vi "WFS Get Spot Dia Statistics.vi"(8 "error in (no error)":errorcluster {"code" format="%.0x"}, 11 "instrument handle":refnum<visa-resource-name>) -> (0 "error out":errorcluster {"code" format="%.0x"}, 1 "Max":dbl, 2 "Min":dbl, 3 "instrument handle out":refnum<visa-resource-name>, 4 "Mean":dbl)   [LabVIEW 2020]
doc: "This VI calculates statistic parameters of the wavefront calculated in WFS Calc Wavefront.vi.\n\nNote: WFS Calc Wavefront.vi is required to run prior to this VI.\nThis VI is not available in Highspeed Mode!"
uses:
  WFS_32.dll
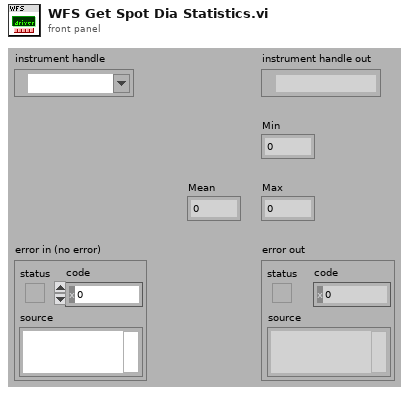
[diagram p1: front panel]
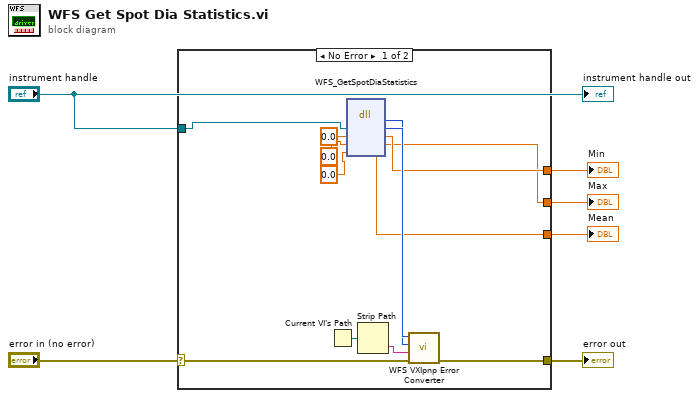
[diagram p0: block diagram]
diagram:
  n1 = case shown="No Error" "error in (no error)" {
    selector: "error in (no error)" -> [w14 w20]
    tunnel: [w13 w20] -> w6
    tunnel: "instrument handle" -> [w18 _]
    tunnel: [w11 _] -> w3
    tunnel: [w9 _] -> w2
    tunnel: [w7 _] -> w1
    frame No Error {
      n2 = Current VI's Path() -> (path=w19:path)
      n3 = dll-call lib="WFS_*.*" fn="WFS_GetSpotDiaStatistics"("Instrument Handle"=w18, "Min"=0.0, "Max"=0.0, "Mean"=0.0) -> (w16:i32, "Instrument Handle"=w17:u32, "Min"=w11:dbl, "Max"=w9:dbl, "Mean"=w7:dbl)  [unwired: 3 in, 2 out]
      n4 = Strip Path(path=w19) -> (name=w15:string)  [unwired: 1 out]
      n5 = call "WFS VXIpnp Error Converter.vi"("error in (no error)"=w14, "Name Of VI (\"\")"=w15, "CVI Error Code (0)"=w16, "instrument handle"=w17) -> ("error out"=w13:errorcluster)  [unwired: 6 in, 1 out]
    }
    frame Error {
    }
  }
  "error out" <- w6
  "Min" <- w3
  "Max" <- w2
  "Mean" <- w1
  "instrument handle out" <- "instrument handle"
